vi "dsp ddc.vi"(7 "reset":bool, 9 "DDC prams":T1 {"frequency shift" format="%#.48g"}, 10 "input valid":bool, 11 "data in":T2) -> (1 "output valid":bool, 2 "number of overflows":u64, 3 "data out":u32)   [LabVIEW 2021]
doc: "Controls whether or not data is written to the DMA FIFO for the acquisition stream. If burst size is 0, this will be a continuous stream, started when the start trigger is asserted. If burst size is greater than zero, acquisition will be in bursts of the designated size, initiated each time the internal state machine is idle and a start trigger is received.\n\nThis VI also keeps track of whether or not an overflow occurred in the acquisition stream and counts the number of overflows that have occurred for debugging information.\n\nThe internal state machine returns the number of samples processed since the most recent acquisition began and the current state machine state."
uses:
  <instrlib>/_niInstr/DSP/v1/Shared/Public/IQ Data.ctl
  <instrlib>/_niInstr/Basic Elements/v1/FPGA/Private/Count Up U8.vi
  <instrlib>/_niInstr/Basic Elements/v1/FPGA/Private/Count Up U64.vi
  <instrlib>/_niInstr/DSP/v1/FPGA/Public/Sub VIs/Frequency Shift/Frequency Shift - 1 spc.vi
  <instrlib>/_niInstr/DSP/v1/FPGA/Public/Sub VIs/Fractional Decimator/Fractional Decimator - 1 spc - 2x oc.vi
  <instrlib>/_niInstr/DSP/v1/FPGA/Public/Sub VIs/Data Conversion/IQ to U32 - 1 spc - S18.1.vi
  <instrlib>/_niInstr/DSP/v1/Xnodes/Public/Decimator/niInstr DSP v1 Decimator FPGA.xnode
  <instrlib>/_niInstr/DSP/v1/FPGA/niInstr DSP v1 FPGA.lvlib
  <instrlib>/_niInstr/Basic Elements/v1/FPGA/niInstr Basic Elements v1 FPGA.lvlib
  <instrlib>/_niInstr/DSP/v1/Shared/niInstr DSP v1 Shared.lvlib
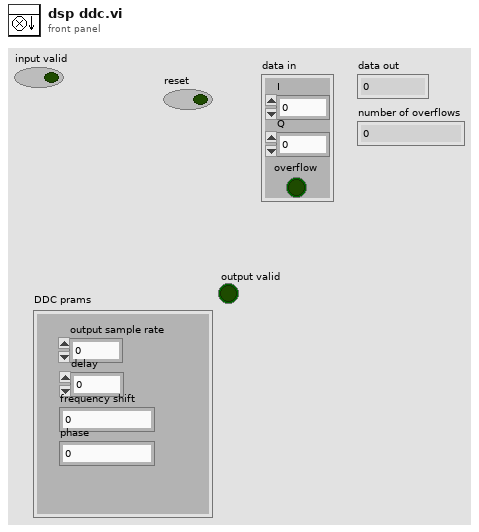
[diagram p1: front panel]
types:
  T1 = cluster{"output sample rate":fxp<+,48,1>, "delay":fxp<+/-,16,0>, "frequency shift":fxp<+/-,48,0>, "phase":fxp<+/-,21,0>}
  T2 = typedef "niInstr DSP v1 Shared.lvlib/IQ Data.ctl" = cluster{"I":fxp<+/-,18,1>, "Q":fxp<+/-,18,1>, "overflow":bool}
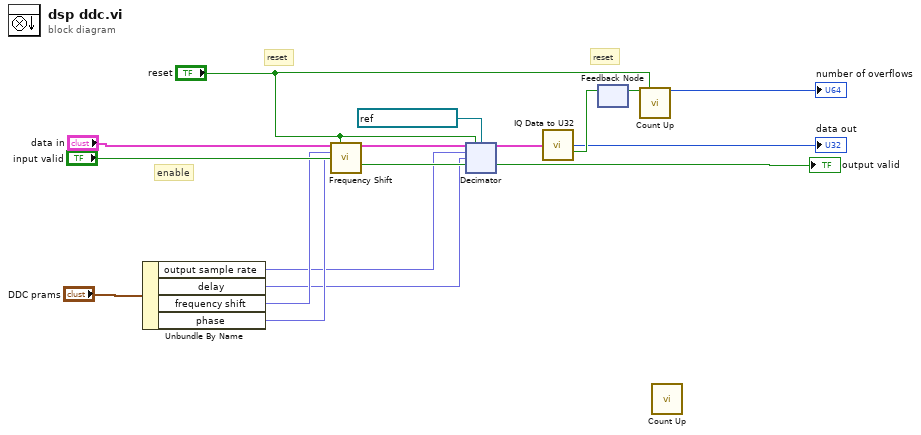
[diagram p0: block diagram]
diagram:
  # "reset"
  # "reset"
  # "enable"
  n1 = Unbundle By Name("DDC prams") -> ("output sample rate"=w2:fxp<+,48,1>, "delay"=w1:fxp<+/-,16,0>, "frequency shift"=w4:fxp<+/-,48,0>, "phase"=w3:fxp<+/-,21,0>)
  n2 = call-poly <instrlib>:"Frequency Shift.vi"("data in"="data in", "reset"="reset", "frequency shift"=w4, "phase"=w3, "input valid"="input valid") -> ("data out"=w13:T2, "output valid"=w10:bool)  [unwired: 7 in, 2 out]
  n3 = xnode "Decimator"("data in"=w13, "reset"="reset", "input valid"=w10, "output sample rate"=w2, "delay"=w1, "clock x2"=refnum<k21> "Data Clock x2" ("oversample clock")) -> ("data out"=w12:T2, "output valid"=→"output valid":bool)  [unwired: 1 out]
  n4 = call-poly <instrlib>:"IQ Data to U32.vi"("IQ data"=w12) -> ("U32 data"=→"data out":u32, "overflow"=w17:bool)  [unwired: 13 in]
  n5 = feedback #1() -> (w16:bool)  [unwired: 1 in]
  n6 = feedback-in #1(w17) -> ()
  n7 = call-poly <instrlib>:"Count Up.vi"("increment"=w16, "reset"="reset") -> ("count out"=→"number of overflows":u64)  [unwired: 13 in]
  n8 = call-poly <instrlib>:"Count Up.vi"() -> ()  [unwired: 15 in, 1 out]
